vi "OP500ZP_ISO.vi"(8 "entrée d'erreur (pas d'erreur)":errorcluster, 9 "Oui":bool, 10 "reference en entrée":refnum<vi>) -> (0 "sortie d'erreur":errorcluster, 3 "Booléen":bool, 4 "ISOP":string, 6 "ISOM":string)   [LabVIEW 2020]
uses:
  VG/PackType.vi
  OP500ZP_VGConf.vi
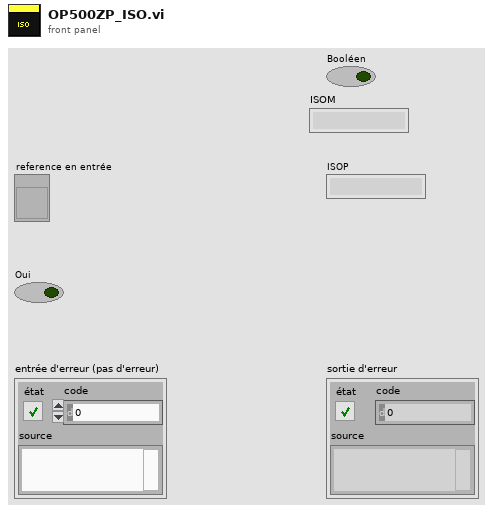
[diagram p1: front panel]
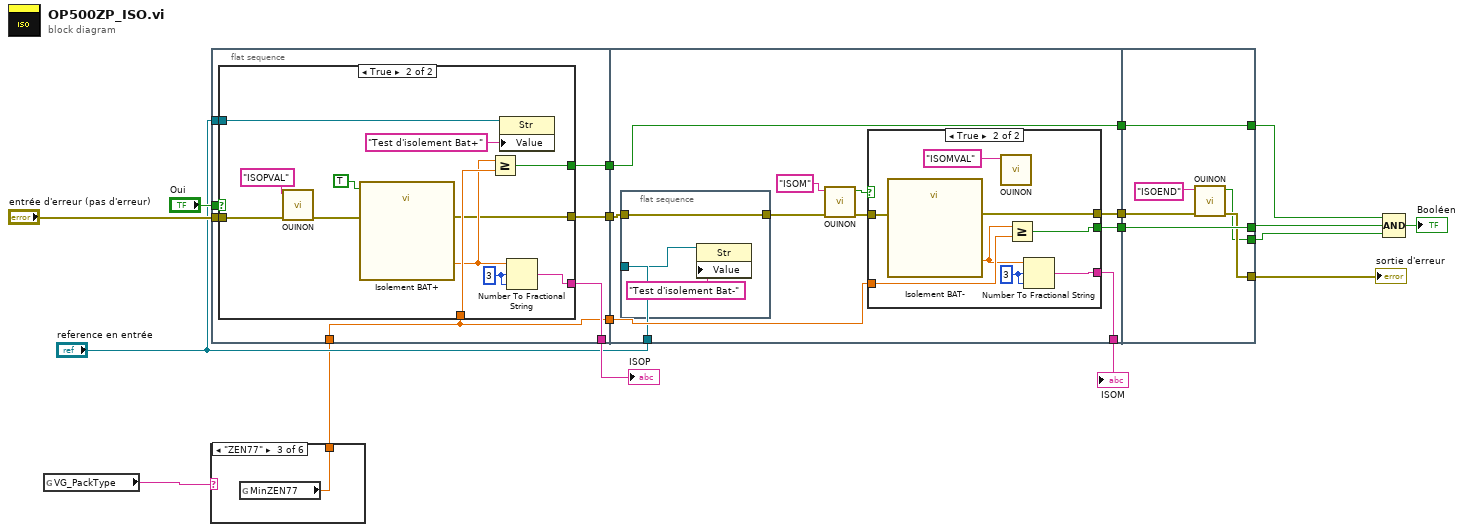
[diagram p0: block diagram]
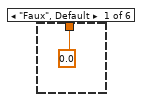
[diagram p2: hidden frame]
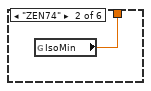
[diagram p3: hidden frame]
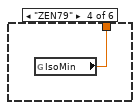
[diagram p4: hidden frame]
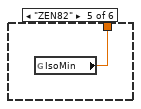
[diagram p5: hidden frame]
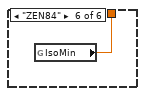
[diagram p6: hidden frame]
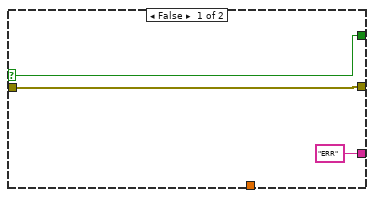
[diagram p7: hidden frame]
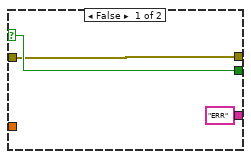
[diagram p8: hidden frame]
diagram:
  n1 = global read "PackType.vi" "VG_PackType"() -> (w3:string)
  n2 = case shown="\"ZEN77\"" w3 {
    tunnel: [0.0 ("IsoMin") w20 w21 w22 w23 w24] -> w2
    frame "Faux", Default {
    }
    frame "ZEN74" {
      n3 = global read "OP500ZP_VGConf.vi" "IsoMin"() -> (w20:dbl)
    }
    frame "ZEN77" {
      n4 = global read "OP500ZP_VGConf.vi" "MinZEN77"() -> (w21:dbl)
    }
    frame "ZEN79" {
      n5 = global read "OP500ZP_VGConf.vi" "IsoMin"() -> (w22:dbl)
    }
    frame "ZEN82" {
      n6 = global read "OP500ZP_VGConf.vi" "IsoMin"() -> (w23:dbl)
    }
    frame "ZEN84" {
      n7 = global read "OP500ZP_VGConf.vi" "IsoMin"() -> (w24:dbl)
    }
  }
  n8 = flat-sequence {
    tunnel: [w25] -> w18
    tunnel: [w31] -> w17
    tunnel: [w30] -> w16
    tunnel: [w29] -> w10
    tunnel: "entrée d'erreur (pas d'erreur)" -> [w28]
    tunnel: "Oui" -> [w27]
    tunnel: "reference en entrée" -> [w26]
    tunnel: w2 -> [w25]
    tunnel: w18 -> [w52]
    tunnel: w17 -> [w57]
    tunnel: w16 -> [w56]
    tunnel: [w57] -> w15
    tunnel: [w51] -> w14
    tunnel: [w50] -> w13
    tunnel: [w49] -> w1
    tunnel: "reference en entrée" -> [w47]
    tunnel: [w76] -> w7
    tunnel: [w77] -> w5
    tunnel: w15 -> [w77]
    tunnel: w14 -> [w72]
    tunnel: w13 -> [w76]
    tunnel: [w75] -> w8
    tunnel: [w74] -> w9
    frame #0 {
      n9 = case shown="True" w27 {
        selector: w27 -> [w33 _]
        tunnel: w28 -> [w34 w36]
        tunnel: [w34 w39] -> w30
        tunnel: ["ERR" w42] -> w29
        tunnel: [w33 w43] -> w31
        tunnel: w25 -> [_ w45]
        tunnel: w26 -> [_ w37]
        frame False {
        }
        frame True {
          w46 = i16 3 ("largeur (-)")
          n10 = call "OUINON.vi"("errin"=w36, "image"="ISOPVAL") -> ("error out"=w35:errorcluster)  [unwired: 8 in, 1 out]
          n11 = call "Isolement BAT+"("Enable"=TRUE, "error in (no error)"=w35) -> ("ISOP"=w44:dbl, "error out"=w39:errorcluster)  [unwired: 15 in, 1 out]
          n12 = Greater Or Equal?(x=w44, y=w45) -> (x >= y?=w43:bool)
          n13 = property class="Str"(reference=w37, "Value"="Test d'isolement Bat+" ("TOP")) -> ()  [unwired: 1 in, 2 out]
          n14 = Number To Fractional String(number=w44, width (-)=w46, precision (6)=w46) -> (F-format string=w42:string)  [unwired: 1 in]
        }
      }
    }
    frame #1 {
      n15 = flat-sequence {
        tunnel: w56 -> [w59]
        tunnel: [w59] -> w55
        tunnel: w47 -> [w58]
        frame #0 {
          n16 = property class="Str"(reference=w58, "Value"="Test d'isolement Bat-" ("TOP")) -> ()  [unwired: 1 in, 2 out]
        }
      }
      n17 = call "OUINON.vi"("errin"=w55, "image"="ISOM" ("IN")) -> ("error out"=w48:errorcluster, "OUI/NON"=w53:bool)  [unwired: 8 in]
      n18 = case shown="True" w53 {
        selector: w53 -> [w63 _]
        tunnel: [w61 w67] -> w51
        tunnel: ["ERR" w64] -> w49
        tunnel: [w63 w68] -> w50
        tunnel: w52 -> [_ w70]
        tunnel: w48 -> [w61 w65]
        frame False {
        }
        frame True {
          w71 = i16 3 ("largeur (-)")
          n19 = call "Isolement BAT-"("error in (no error)"=w65) -> ("ISOM"=w69:dbl, "error out"=w67:errorcluster)  [unwired: 16 in, 1 out]
          n20 = call "OUINON.vi"("image"="ISOMVAL") -> ()  [unwired: 9 in, 2 out]
          n21 = Greater Or Equal?(x=w69, y=w70) -> (x >= y?=w68:bool)
          n22 = Number To Fractional String(number=w69, width (-)=w71, precision (6)=w71) -> (F-format string=w64:string)  [unwired: 1 in]
        }
      }
    }
    frame #2 {
      n23 = call "OUINON.vi"("errin"=w72, "image"="ISOEND") -> ("error out"=w75:errorcluster, "OUI/NON"=w74:bool)  [unwired: 8 in]
    }
  }
  n24 = Compound Arithmetic op=AND ("Opérateur arithmétique")(w5, w7, w9) -> (→"Booléen":bool)
  "ISOP" <- w10
  "sortie d'erreur" <- w8
  "ISOM" <- w1
